vi "Check UART Pins.vi"(8 "error in (no error)":errorcluster, 9 "UART Pins":T2={"TX GPIO"=-1, "RX GPIO"=-1}, 10 "UART #":T1=-1, 11 "Session in":refnum<class "Session.lvclass">) -> (0 "error out":errorcluster, 3 "Session out":refnum<class "Session.lvclass">)   [LabVIEW 2024, in "CTI.lvlib" / "Session.lvclass"]
uses:
  Session.lvclass
  UART Pins.ctl
  GPIO Number.ctl
  UART Number.ctl
  Session.lvclass/Session.ctl
  CTI.lvlib
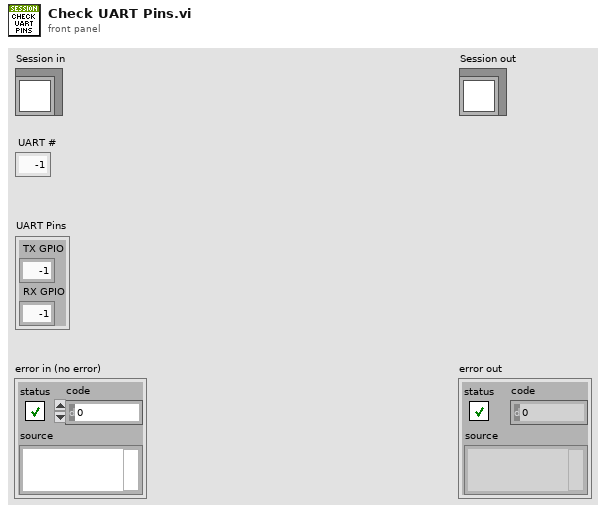
[diagram p1: front panel]
types:
  T1 = typedef "CTI.lvlib/UART Number.ctl" = i8
  T2 = typedef "CTI.lvlib/UART Pins.ctl" = cluster{"TX GPIO":T3, "RX GPIO":T3}
  T3 = typedef "CTI.lvlib/GPIO Number.ctl" = i8
  T4 = typedef "CTI.lvlib/Available UART.ctl" = cluster{"UART #":T1, "TX GPIOs":T3[], "RX GPIOs":T3[]}
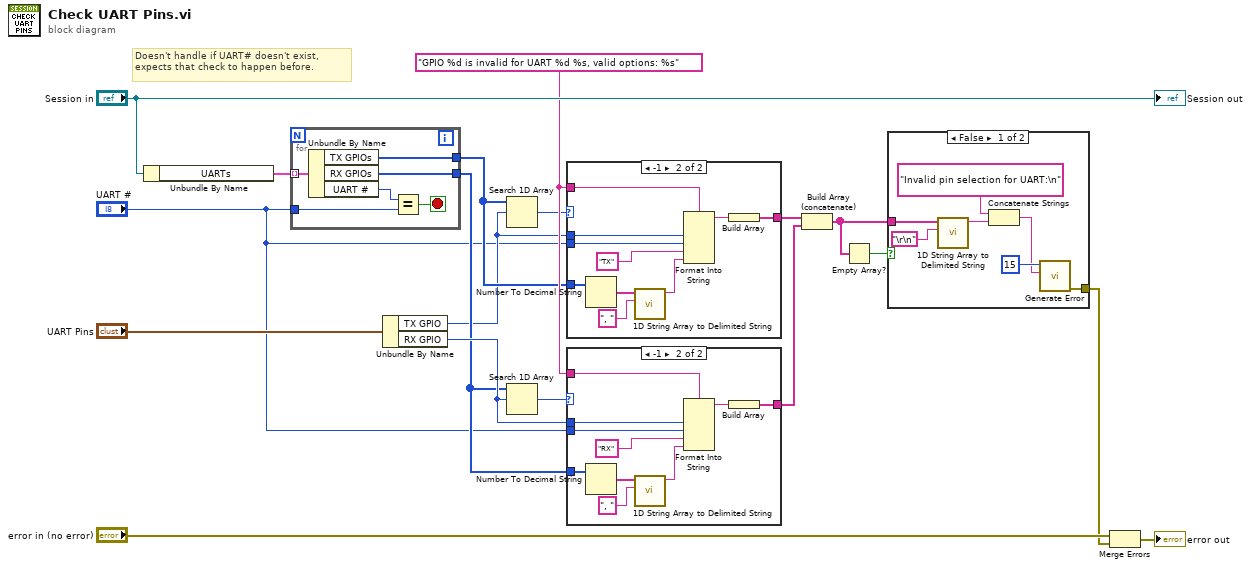
[diagram p0: block diagram]
diagram:
  w11 = "GPIO %d is invalid for UART %d %s, valid options: %s"
  # "Doesn't handle if UART# doesn't exist, expects that check to happen before."
  n1 = Unbundle By Name("Session in") -> ("UARTs"=w15:T4[])
  n2 = for {
    tunnel: w15 -> [w24] mode=indexing
    tunnel: "UART #" -> [w23]
    tunnel: [w21] -> w9
    tunnel: [w20] -> w12
    stop <- w19 stop-if-true
    n3 = Unbundle By Name(w24) -> ("TX GPIOs"=w21:T3[], "RX GPIOs"=w20:T3[], "UART #"=w22:T1)
    n4 = Equal?(x=w22, y=w23) -> (x = y?=w19:bool)
  }
  n5 = Unbundle By Name("UART Pins") -> ("TX GPIO"=w8:T3, "RX GPIO"=w13:T3)
  n6 = Search 1D Array(1D array=w9, element=w8) -> (index of element=w10:i32)  [unwired: 1 in]
  n7 = Search 1D Array(1D array=w12, element=w13) -> (index of element=w14:i32)  [unwired: 1 in]
  n8 = case shown="-1" w10 {
    tunnel: w11 -> [_ w34]
    tunnel: "UART #" -> [_ w32]
    tunnel: w8 -> [_ w33]
    tunnel: w9 -> [_ w30]
    tunnel: [_ w25] -> w6
    frame Default {
    }
    frame -1 {
      n9 = Number To Decimal String(number=w30) -> (decimal integer string=w29:string[])  [unwired: 1 in]
      n10 = call <vilib>:"1D String Array to Delimited String.vi"("delimiter"=", ", "string array"=w29) -> ("delimited string"=w27:string)  [unwired: 9 in]
      n11 = Format Into String(format string=w34, w33, w32, "TX" ("input 3"), w27) -> (resulting string=w26:string)  [unwired: 2 in, 1 out]
      n12 = Build Array(w26) -> (w25:string[])
    }
  }
  n13 = case shown="-1" w14 {
    tunnel: w11 -> [_ w44]
    tunnel: "UART #" -> [_ w42]
    tunnel: w13 -> [_ w43]
    tunnel: w12 -> [_ w40]
    tunnel: [_ w35] -> w5
    frame Default {
    }
    frame -1 {
      n14 = Number To Decimal String(number=w40) -> (decimal integer string=w39:string[])  [unwired: 1 in]
      n15 = call <vilib>:"1D String Array to Delimited String.vi"("delimiter"=", ", "string array"=w39) -> ("delimited string"=w37:string)  [unwired: 9 in]
      n16 = Format Into String(format string=w44, w43, w42, "RX" ("input 3"), w37) -> (resulting string=w36:string)  [unwired: 2 in, 1 out]
      n17 = Build Array(w36) -> (w35:string[])
    }
  }
  n18 = Build Array (concatenate)(w6, w5) -> (w3:string[])
  n19 = Empty Array?(array=w3) -> (empty?=w4:bool)
  n20 = case shown="False" w4 {
    tunnel: w3 -> [w51 _]
    tunnel: [w48 _] -> w1
    frame False {
      n21 = call <vilib>:"1D String Array to Delimited String.vi"("delimiter"="\r\n", "string array"=w51) -> ("delimited string"=w46:string)  [unwired: 9 in]
      n22 = Concatenate Strings("Invalid pin selection for UART:\n" ("format string"), w46) -> (w45:string)
      n23 = call "Generate Error.vi"("error message"=w45, "error code"=15) -> ("error out"=w48:errorcluster)  [unwired: 9 in]
    }
    frame True {
    }
  }
  n24 = Merge Errors("error in (no error)", w1) -> (→"error out":errorcluster)
  "Session out" <- "Session in"
